vi "Simple waveform generator.vi"() -> ()   [LabVIEW 2020]
uses:
  <vilib>/measure/NI_MABase.lvlib
panel:
  in  "frequency 2":dbl=10.0 format="%0.2p"
  out "Waveform Chart 2":waveform(dbl)(graph)
  in  "stop 4":bool
  in  "stop 3":bool
  out "Waveform Chart":waveform(dbl)(graph)
  in  "frequency":dbl=10.0 format="%0.2p"
  in  "stop 2":bool
  in  "stop":bool
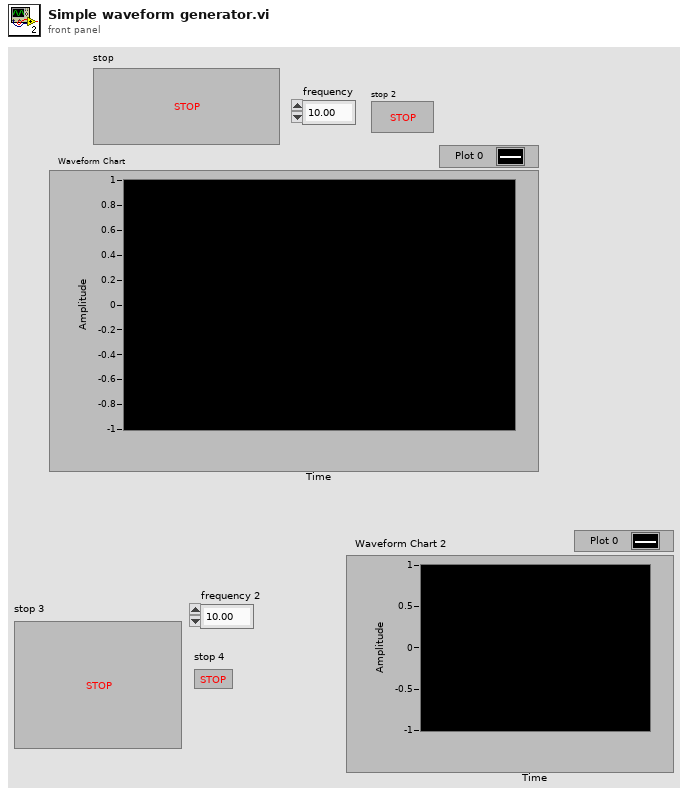
[diagram p1: front panel]
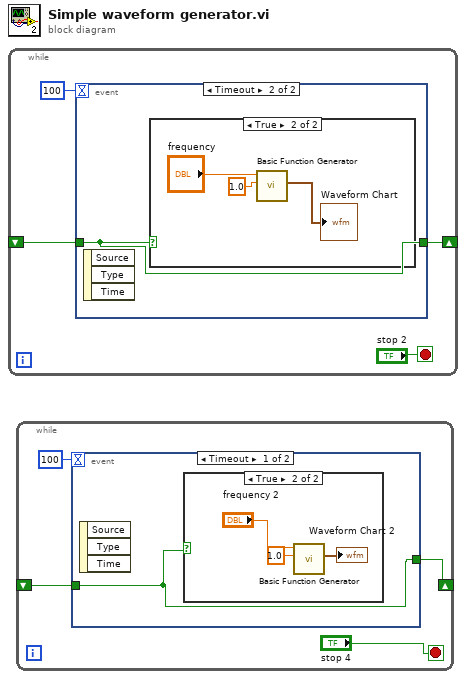
[diagram p0: block diagram]
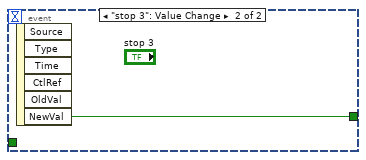
[diagram p3: hidden frame]
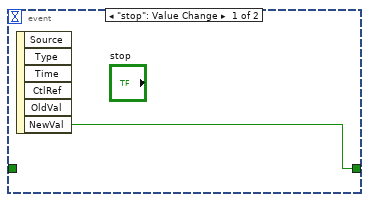
[diagram p4: hidden frame]
diagram:
  n1 = while {
    shift-right: [w2] -> _
    shift-left: _ -> [w1]
    stop <- "stop 2" stop-if-true
    n2 = event shown="[1] Timeout" {
      selector: _ -> [_ _]
      dyn-events: _ -> [_ _]
      timeout: 100 -> [_ _]
      tunnel: [w5 w6] -> w2
      tunnel: w1 -> [_ w6]
      event "stop": Value Change {
        n3 = event-data() -> ("NewVal"=w5:bool)  [unwired: 1 in, 5 out]
      }
      event Timeout {
        n4 = event-data() -> ()  [unwired: 1 in, 3 out]
        n5 = case shown="True" w6 {
          frame False {
          }
          frame True {
            n6 = call <vilib>:"Basic Function Generator.vi"("amplitude"=1.0, "frequency"="frequency") -> ("signal out"=→"Waveform Chart":waveform(dbl))  [unwired: 7 in, 2 out]
          }
        }
      }
    }
  }
  n7 = while {
    shift-right: [w10] -> _
    shift-left: _ -> [w11]
    stop <- "stop 4" stop-if-true
    n8 = event shown="[0] Timeout" {
      selector: _ -> [_ _]
      dyn-events: _ -> [_ _]
      timeout: 100 -> [_ _]
      tunnel: w11 -> [w14 _]
      tunnel: [w14 w18] -> w10
      event Timeout {
        n9 = event-data() -> ()  [unwired: 1 in, 3 out]
        n10 = case shown="True" w14 {
          frame False {
          }
          frame True {
            n11 = call <vilib>:"Basic Function Generator.vi"("amplitude"=1.0, "frequency"="frequency 2") -> ("signal out"=→"Waveform Chart 2":waveform(dbl))  [unwired: 7 in, 2 out]
          }
        }
      }
      event "stop 3": Value Change {
        n12 = event-data() -> ("NewVal"=w18:bool)  [unwired: 1 in, 5 out]
      }
    }
  }
